vi "BRig_RT__Case_Exp__recordLick.vi"(0 "input_dataLick":u16[][](array[numeric]), 1 "input_lick__R":bool, 2 "input_lick__L":bool, 3 "input_lick":bool, 9 "intput_state__trialStart":T1, 11 "intput_state__trialEnd":T1, 12 "input_dataCurrent":u16[](array[numeric])) -> (4 "output_dataLick":u16[][](array[numeric]), 14 "output_dataCurrent":u16[](array[numeric]))   [LabVIEW 2014]
uses:
  myRIO_BRig_RT__Case_Exp_stateList.ctl
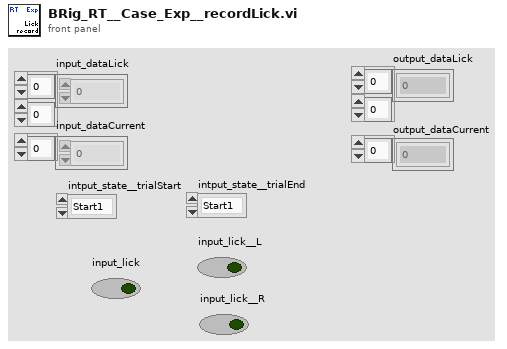
[diagram p1: front panel]
types:
  T1 = typedef "myRIO_BRig_RT__Case_Exp_stateList.ctl" = enum16{"Start1", "Start2", "Start3", "saveSettings1", "saveSettings2", "saveSettings3", "saveSettings4", "saveSettings_LC_ENL_l1", "saveSettings_LC_ENL_l2", "saveSettings_LC_Cue_l1", "saveSettings_LC_Cue_l2", "saveSettings6_LC_l1_Other", "SaveSettings6_LC_l2_Other", "setSettings_Audio", "setSettings_Laser", "initBlock_pre", "initBlock", "initBlock2", "initBlock_post", "initTrial_pre", "initTrial", "initTrial2", "initTrial3", "initTrial4", "initTrial_LC_ENL1", "initTrial_LC_Cue1", "initTrial_LC_Cue1_2", "initTrial_LC_Sel", "initTrial_post", "ENL1_pre", "ENL1", "ENL1_post", "ENL1Penalty_pre", "ENL1Penalty", "ENL2_pre", "ENL2", "ENL2Penalty_pre", "ENL2Penalty", "Cue1_pre", "Cue1", "Cue1_post", "Cue1Penalty_pre", "Cue1Penalty", "Cue2_pre", "Cue2", "Cue2Penalty_pre", "Cue2Penalty", "Selection_pre", "Selection", "Select_post", "SelectReward_pre", "SelectReward", "SelectRewardPost_pre", "SelectRewardPost", "SelectWrong_pre", "SelectWrong", "SelectWrong_post", "SelectTimeout_pre", "SelectTimeout", "SelectTimeout_post", "endTrial_pre", "endTrial1", "endTrial2", "endTrial3", "endTrial_post", "endBlock_pre", "endBlock", "endBlock_post", "endExp", "commConnect", "commUpload_pre", "commUpload_dataBlock", "commUpload_dataCurrent", "commUpload_dataExp", "commUpload_dataLC", "commUpload_dataTrial", "commUpload_post", "saveData_pre", "saveData_dataBlock", "saveData_dataCurrent", "saveData_dataExp", "saveData_dataLC", "saveData_dataTrial", "saveData_post", "empty_endBlock1", "empty_endBlock2", "empty_endTrial1", "empty_endTrial2", "empty_endTrial3", "empty_endTrial4", "empty_endTrial5", "dummyState", "dummyState_endBlock", "FreeReward_pre", "FreeReward", "FreeRewardPost_pre", "FreeRewardPost"}
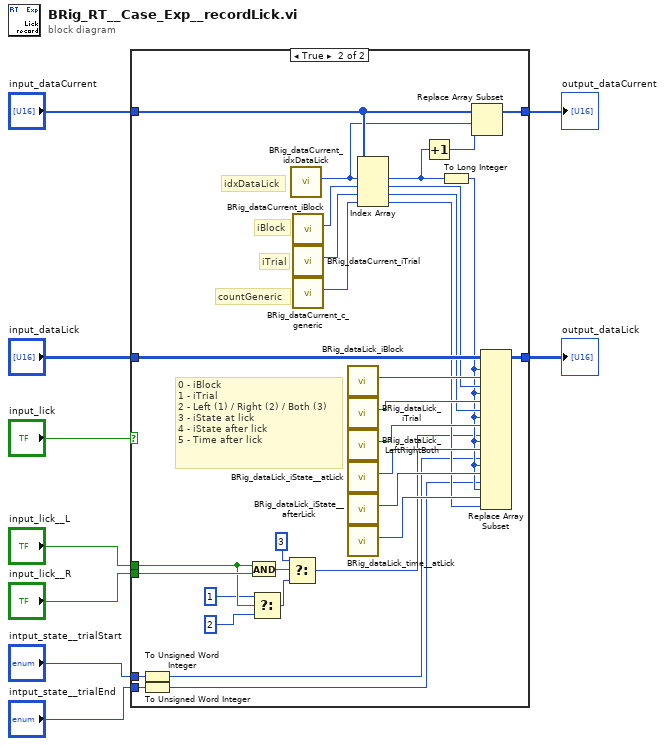
[diagram p0: block diagram]
diagram:
  n1 = case shown="True" "input_lick" {
    tunnel: [w10 w43] -> w9
    tunnel: "input_dataLick" -> [w10 w42]
    tunnel: "input_dataCurrent" -> [w11 w38]
    tunnel: [w11 w35] -> w6
    tunnel: "input_lick__R" -> [_ w21]
    tunnel: "input_lick__L" -> [_ w20]
    tunnel: "intput_state__trialEnd" -> [_ w13]
    tunnel: "intput_state__trialStart" -> [_ w12]
    frame False {
    }
    frame True {
      # "0 - iBlock\n1 - iTrial\n2 - Left (1) / Right (2) / Both (3)\n3 - iState at lick\n4 - iState after lick\n5 - Time after lick"
      # "idxDataLick"
      # "countGeneric"
      # "iTrial"
      # "iBlock"
      n2 = To Unsigned Word Integer(number=w12) -> (unsigned 16bit integer=w15:u16)
      n3 = To Unsigned Word Integer(number=w13) -> (unsigned 16bit integer=w14:u16)
      n4 = And(x=w20, y=w21) -> (x .and. y?=w25:bool)
      n5 = Select(t=u16 1, s=w20, f=u16 2) -> (s? t:f=w17:u16)
      n6 = Select(t=u16 3, s=w25, f=w17) -> (s? t:f=w16:u16)
      n7 = call "BRig_dataCurrent_idxDataLick.vi"() -> ("output_idxDataLick"=w37:i32)  [unwired: 11 in]
      n8 = call "BRig_dataCurrent_iBlock.vi"() -> ("output_iBlock"=w39:i32)  [unwired: 11 in]
      n9 = call "BRig_dataCurrent_iTrial.vi"() -> ("output_iTrial"=w40:i32)  [unwired: 11 in]
      n10 = call "BRig_dataCurrent_c_generic.vi"() -> ("output_count_generic"=w41:i32)  [unwired: 11 in]
      n11 = call "BRig_dataLick_iBlock.vi"() -> ("output_iBlock"=w34:i32)  [unwired: 11 in]
      n12 = call "BRig_dataLick_iTrial.vi"() -> ("output_iTrial"=w32:i32)  [unwired: 11 in]
      n13 = call "BRig_dataLick_LeftRightBoth.vi"() -> ("output_LeftRightBoth"=w30:i32)  [unwired: 11 in]
      n14 = call "BRig_dataLick_iState__atLick.vi"() -> ("output_iState__atLick"=w29:i32)  [unwired: 11 in]
      n15 = call "BRig_dataLick_iState__afterLick.vi"() -> ("output_iState__afterLick"=w28:i32)  [unwired: 11 in]
      n16 = call "BRig_dataLick_time__atLick.vi"() -> ("output_time__atLick"=w27:i32)  [unwired: 11 in]
      n17 = Index Array(array=w38, index #1=w37, index #2=w39, index #3=w40, index #4=w41) -> (element #1=w24:u16, element #2=w33:u16, element #3=w31:u16, element #4=w26:u16)
      n18 = Increment(x=w24) -> (x+1=w36:u16)
      n19 = To Long Integer(number=w24) -> (32bit integer=w23:i32)
      n20 = Replace Array Subset(array=w38, new element=w36, index=w37) -> (w35:u16[])
      n21 = Replace Array Subset(array=w42, new element #1=w33, index (row) #1=w23, index (col) #1=w34, new element #2=w31, index (row) #2=w23, index (col) #2=w32, new element #3=w16, index (row) #3=w23, index (col) #3=w30, new element #4=w15, index (row) #4=w23, index (col) #4=w29, new element #5=w14, index (row) #5=w23, index (col) #5=w28, new element #6=w26, index (row) #6=w23, index (col) #6=w27) -> (w43:u16[][])
    }
  }
  "output_dataLick" <- w9
  "output_dataCurrent" <- w6
